vi "economizer exv valves.vi"(0 "Coarse Gas Input Cluster":T5={"Hot Gas Bypass\n Coarse Adjust"=100.0, "Accept Autotune Coarse Gas"=FALSE, "Coarse slide in P"=refnum, "file for Coarse gas"=path "", "autotune? Coarse gas"=FALSE, "PID gains in Coarse gas"={"proportional gain (Kc)"=0.0, "integral time (Ti, min)"=0.0, "derivative time (Td, min)"=0.0}} {"Hot Gas Bypass\n Coarse Adjust" min=0.0 max=100.0 step=1.0 scale=0.0..100.0}, 1 "Fine Gas Input Cluster":T6={"Hot Gas Bypass\n Fine Adjust"=100.0, "Accept Autotune Fine Gas"=FALSE, "Fine slide in P"=refnum, "file for fine gas"=path "", "autotune? fine gas"=FALSE, "PID gains in fine gas"={"proportional gain (Kc)"=0.0, "integral time (Ti, min)"=0.0, "derivative time (Td, min)"=0.0}} {"Hot Gas Bypass\n Fine Adjust" min=0.0 max=100.0 step=1.0 scale=0.0..100.0}, 3 "Intermediate T Threshold":dbl=5.0 format="%#_13g", 4 "Intermediate P Threshold":dbl=10.0 format="%#_13g", 5 "Coarse Liq Input Cluster":T3={"Liquid\n Coarse Adjust"=100.0, "Accept Autotune Coarse Liq"=FALSE, "Coarse slide in T"=refnum, "file for Coarse liq"=path "", "autotune? Coarse gas"=FALSE, "PID gains in Coarse Liq"={"proportional gain (Kc)"=0.0, "integral time (Ti, min)"=0.0, "derivative time (Td, min)"=0.0}} {"Liquid\n Coarse Adjust" min=0.0 max=100.0 step=1.0 scale=0.0..100.0}, 7 "Fine Liq Input Cluster":T4={"Liquid\n Fine Adjust"=100.0, "Accept Autotune Fine Liq"=FALSE, "Fine slide in T"=refnum, "file for fine liq"=path "", "autotune? fine liq"=FALSE, "PID gains in fine liq"={"proportional gain (Kc)"=0.0, "integral time (Ti, min)"=0.0, "derivative time (Td, min)"=0.0}} {"Liquid\n Fine Adjust" min=0.0 max=100.0 step=1.0 scale=0.0..100.0}, 8 "Controller Toggle P 2":bool, 9 "Reinitialize Controller P 2":bool, 10 "Economizer ?":bool, 12 "Current Intermediate T":dbl format="%#_13g", 13 "Desired Intermediate T":dbl, 14 "Desired Intermediate P":dbl, 15 "Current Intermediate P":dbl format="%#_13g", 16 "Controller Toggle T 2":bool, 17 "Reinitialize Controller T 2":bool) -> (20 "Gas Valves Output":T2, 27 "Liq Valves Output":T1)   [LabVIEW 2017]
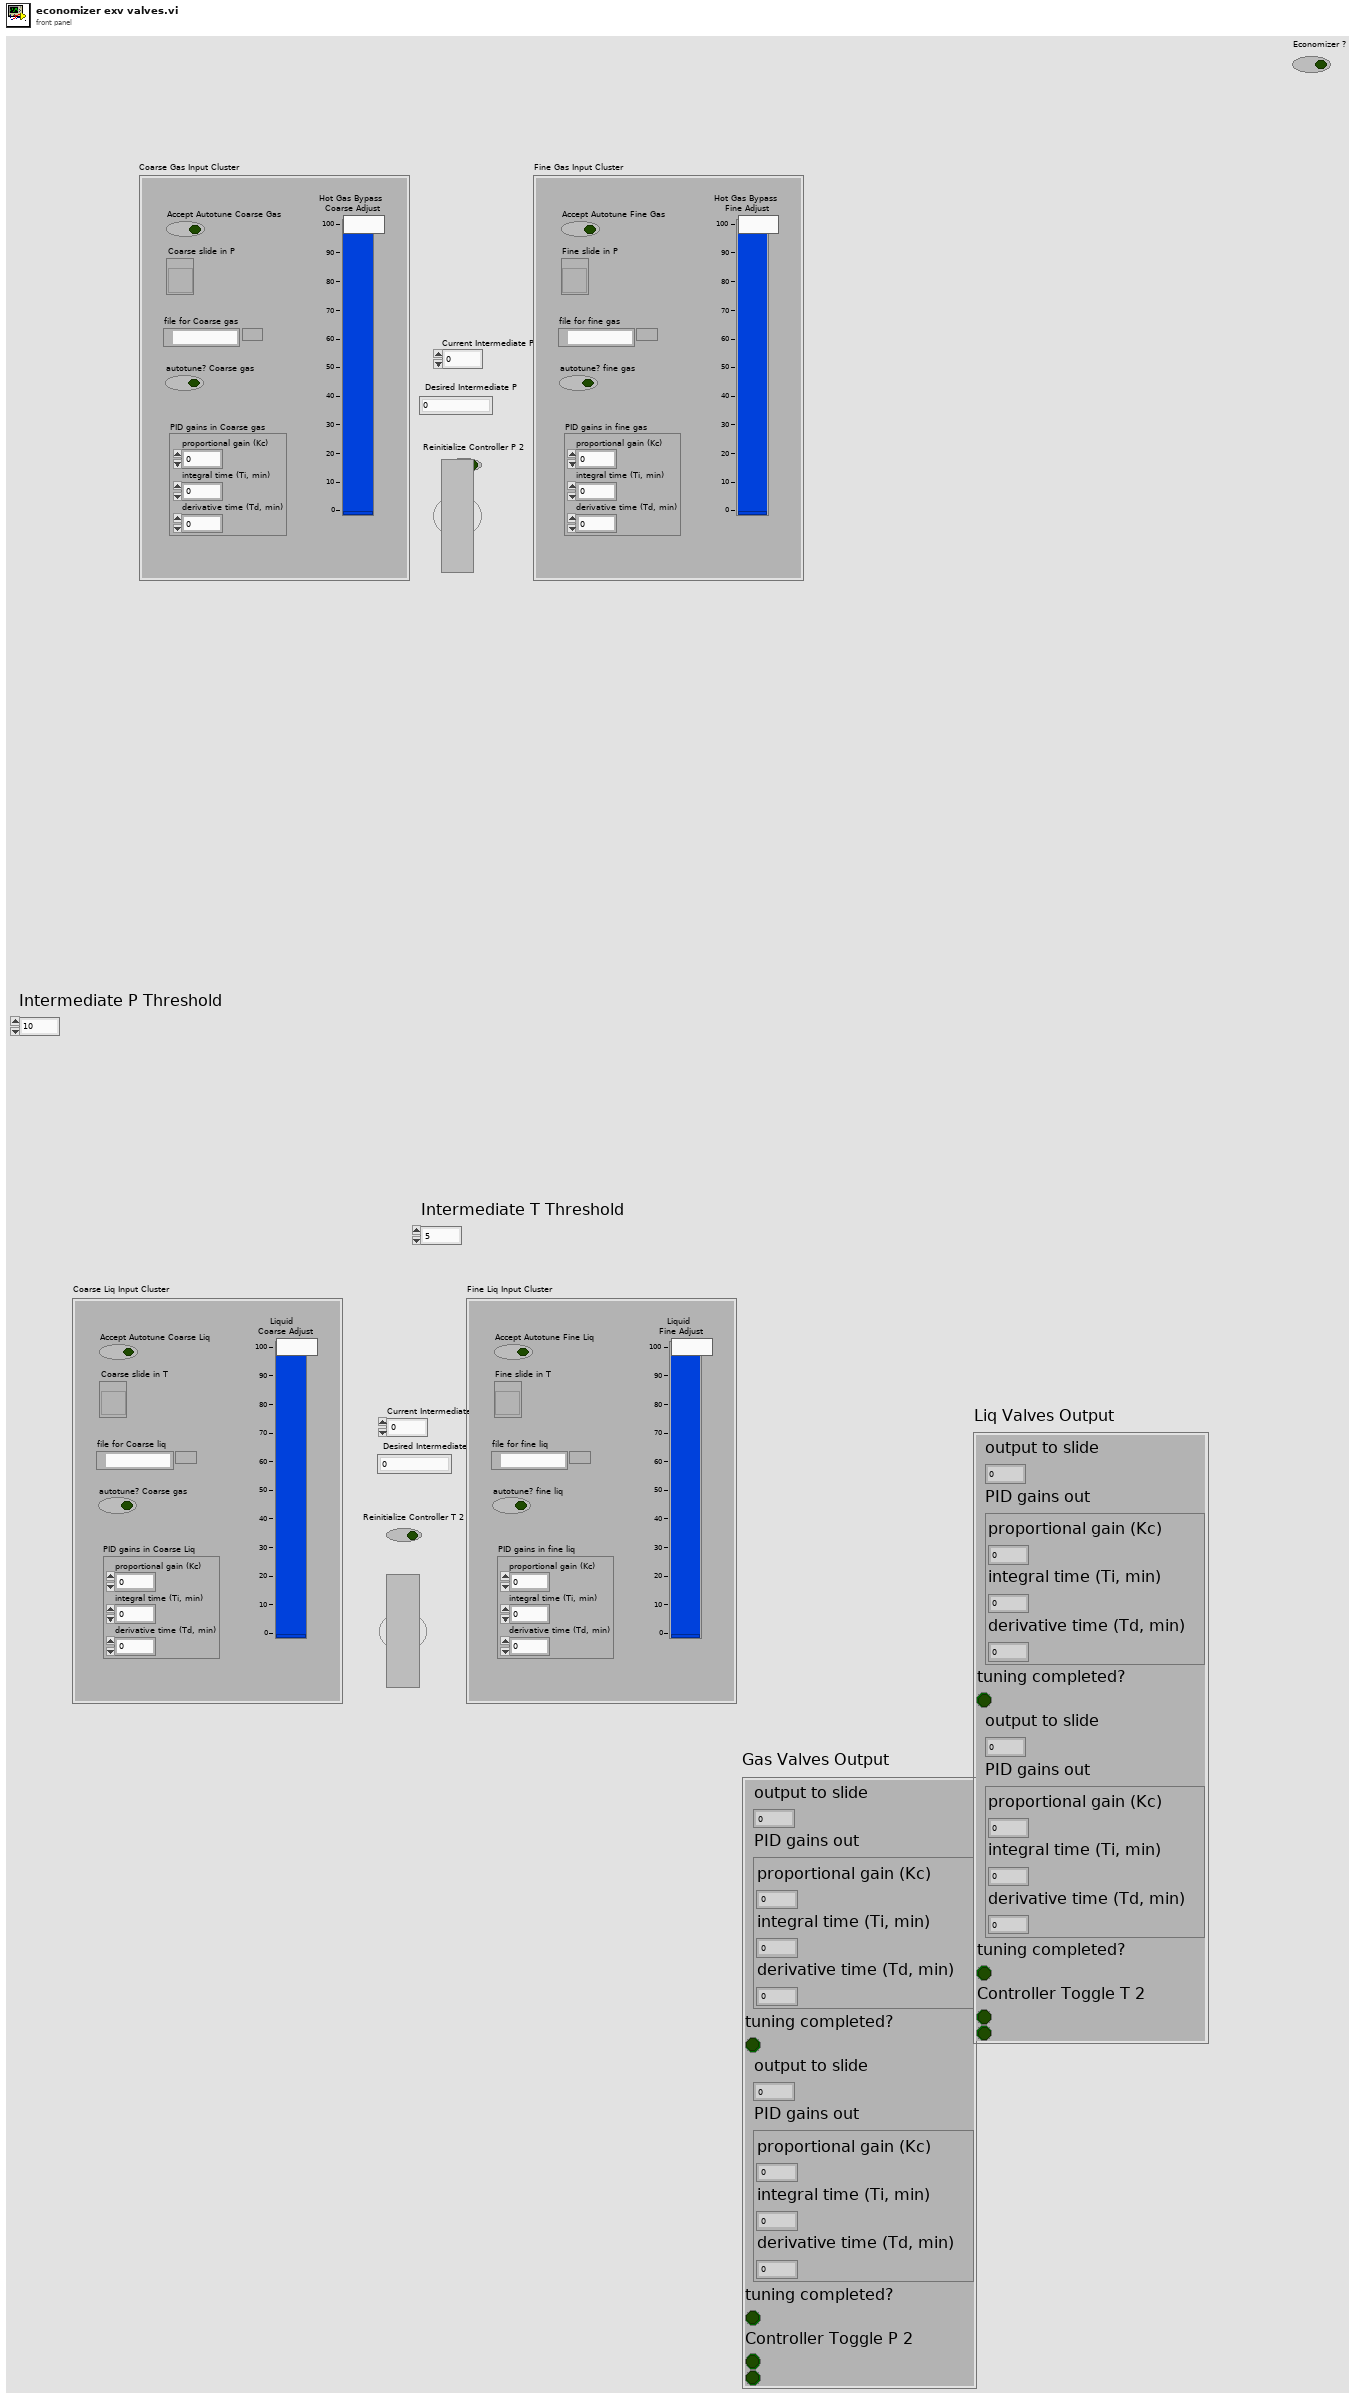
[diagram p1: front panel]
types:
  T1 = cluster{"output to slide":dbl, "PID gains out":cluster{"proportional gain (Kc)":dbl, "integral time (Ti, min)":dbl, "derivative time (Td, min)":dbl}, "tuning completed?":bool, "output to slide":dbl, "PID gains out":cluster{"proportional gain (Kc)":dbl, "integral time (Ti, min)":dbl, "derivative time (Td, min)":dbl}, "tuning completed?":bool, "Controller Toggle T 2":bool, bool}
  T2 = cluster{"output to slide":dbl, "PID gains out":cluster{"proportional gain (Kc)":dbl, "integral time (Ti, min)":dbl, "derivative time (Td, min)":dbl}, "tuning completed?":bool, "output to slide":dbl, "PID gains out":cluster{"proportional gain (Kc)":dbl, "integral time (Ti, min)":dbl, "derivative time (Td, min)":dbl}, "tuning completed?":bool, "Controller Toggle P 2":bool, bool}
  T3 = cluster{"Liquid\n Coarse Adjust":dbl, "Accept Autotune Coarse Liq":bool, "Coarse slide in T":refnum<vi>, "file for Coarse liq":path, "autotune? Coarse gas":bool, "PID gains in Coarse Liq":cluster{"proportional gain (Kc)":dbl, "integral time (Ti, min)":dbl, "derivative time (Td, min)":dbl}}
  T4 = cluster{"Liquid\n Fine Adjust":dbl, "Accept Autotune Fine Liq":bool, "Fine slide in T":refnum<vi>, "file for fine liq":path, "autotune? fine liq":bool, "PID gains in fine liq":cluster{"proportional gain (Kc)":dbl, "integral time (Ti, min)":dbl, "derivative time (Td, min)":dbl}}
  T5 = cluster{"Hot Gas Bypass\n Coarse Adjust":dbl, "Accept Autotune Coarse Gas":bool, "Coarse slide in P":refnum<vi>, "file for Coarse gas":path, "autotune? Coarse gas":bool, "PID gains in Coarse gas":cluster{"proportional gain (Kc)":dbl, "integral time (Ti, min)":dbl, "derivative time (Td, min)":dbl}}
  T6 = cluster{"Hot Gas Bypass\n Fine Adjust":dbl, "Accept Autotune Fine Gas":bool, "Fine slide in P":refnum<vi>, "file for fine gas":path, "autotune? fine gas":bool, "PID gains in fine gas":cluster{"proportional gain (Kc)":dbl, "integral time (Ti, min)":dbl, "derivative time (Td, min)":dbl}}
  T7 = cluster{"proportional gain (Kc)":dbl, "integral time (Ti, min)":dbl, "derivative time (Td, min)":dbl}
  T8 = enum8{"Enabled", "Disabled", "Disabled and Grayed Out"}
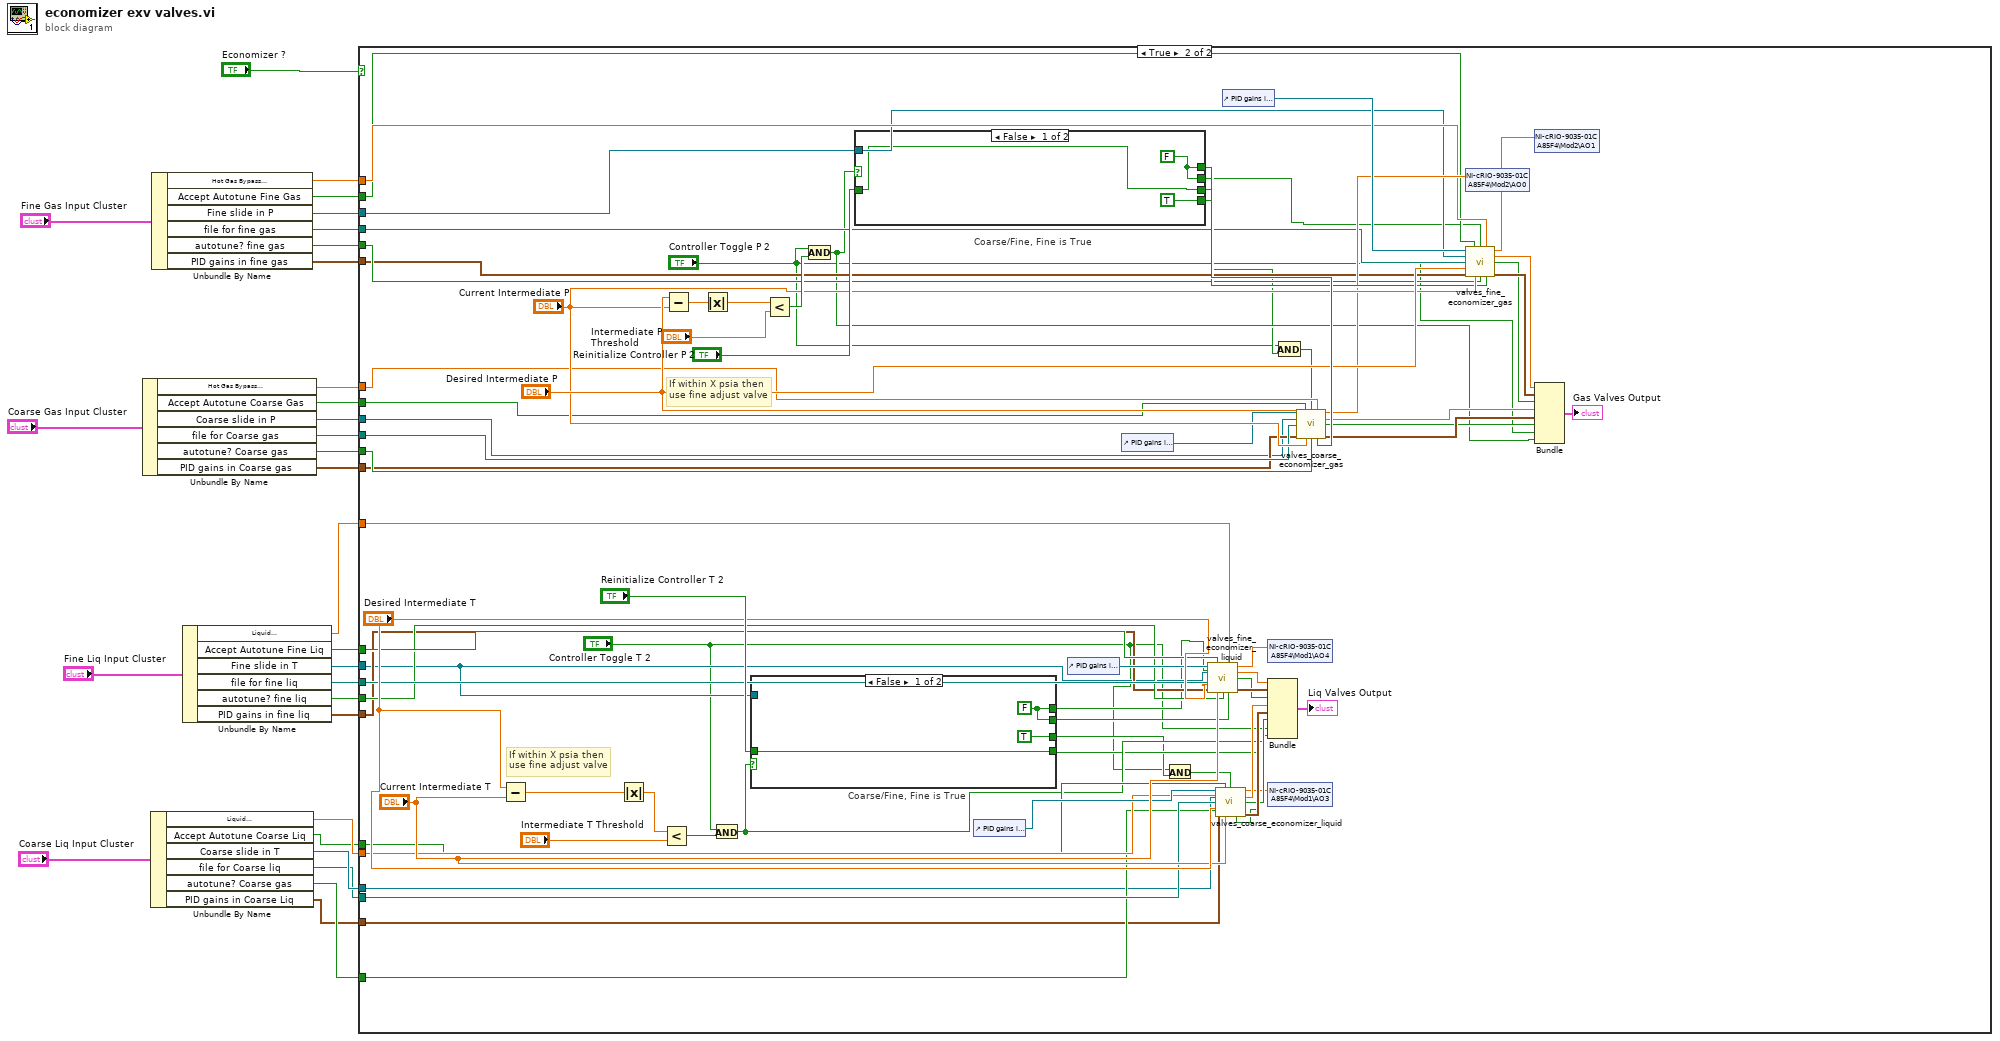
[diagram p0: block diagram]
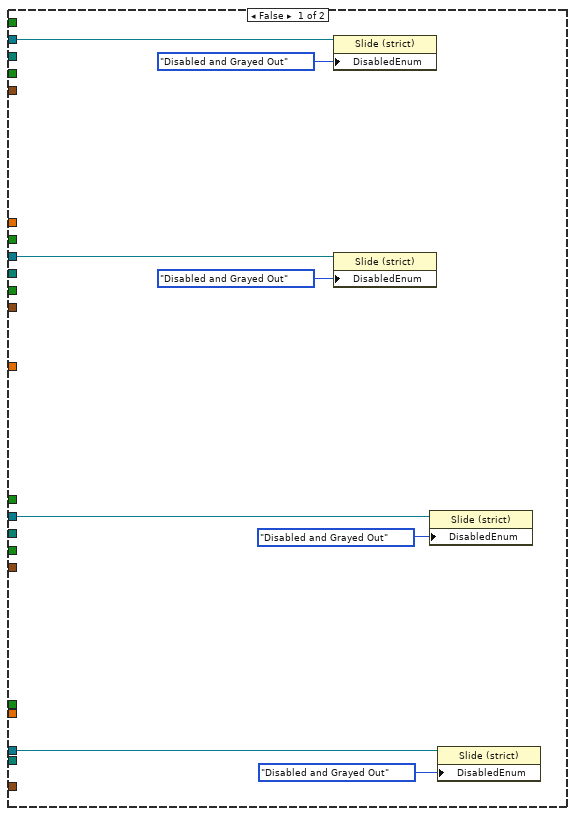
[diagram p2: hidden frame]
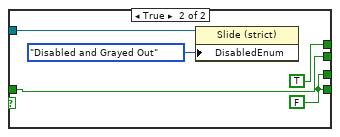
[diagram p3: hidden frame]
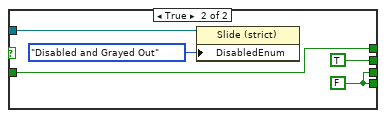
[diagram p4: hidden frame]
diagram:
  n1 = Unbundle By Name("Coarse Gas Input Cluster") -> ("Hot Gas Bypass\n Coarse Adjust"=w21:dbl, "Accept Autotune Coarse Gas"=w20:bool, "Coarse slide in P"=w19:refnum<vi>, "file for Coarse gas"=w18:path, "autotune? Coarse gas"=w17:bool, "PID gains in Coarse gas"=w16:T7)
  n2 = Unbundle By Name("Coarse Liq Input Cluster") -> ("Liquid\n Coarse Adjust"=w7:dbl, "Accept Autotune Coarse Liq"=w6:bool, "Coarse slide in T"=w5:refnum<vi>, "file for Coarse liq"=w4:path, "autotune? Coarse gas"=w3:bool, "PID gains in Coarse Liq"=w2:T7)
  n3 = Unbundle By Name("Fine Gas Input Cluster") -> ("Hot Gas Bypass\n Fine Adjust"=w28:dbl, "Accept Autotune Fine Gas"=w27:bool, "Fine slide in P"=w26:refnum<vi>, "file for fine gas"=w25:path, "autotune? fine gas"=w24:bool, "PID gains in fine gas"=w23:T7)
  n4 = Unbundle By Name("Fine Liq Input Cluster") -> ("Liquid\n Fine Adjust"=w14:dbl, "Accept Autotune Fine Liq"=w13:bool, "Fine slide in T"=w12:refnum<vi>, "file for fine liq"=w11:path, "autotune? fine liq"=w10:bool, "PID gains in fine liq"=w9:T7)
  n5 = case shown="True" "Economizer ?" {
    tunnel: w28 -> [_ w92]
    tunnel: w27 -> [_ w91]
    tunnel: w26 -> [w36 w47]
    tunnel: w25 -> [_ w90]
    tunnel: w24 -> [_ w89]
    tunnel: w23 -> [_ w88]
    tunnel: w21 -> [_ w87]
    tunnel: w20 -> [_ w86]
    tunnel: w19 -> [w34 w53]
    tunnel: w18 -> [_ w85]
    tunnel: w17 -> [_ w84]
    tunnel: w16 -> [_ w83]
    tunnel: w14 -> [_ w66]
    tunnel: w13 -> [_ w65]
    tunnel: w12 -> [w31 w48]
    tunnel: w11 -> [_ w64]
    tunnel: w10 -> [_ w63]
    tunnel: w9 -> [_ w62]
    tunnel: w7 -> [_ w61]
    tunnel: w6 -> [_ w60]
    tunnel: w5 -> [w30 w54]
    tunnel: w4 -> [_ w59]
    tunnel: w3 -> [_ w58]
    tunnel: w2 -> [_ w57]
    frame False {
      n6 = property on="Property Node" class="Slide (strict)"(reference=w36, "DisabledEnum"=T8."Disabled and Grayed Out" ("Disabled")) -> ()  [unwired: 1 in, 2 out]
      n7 = property on="Property Node" class="Slide (strict)"(reference=w34, "DisabledEnum"=T8."Disabled and Grayed Out" ("Disabled")) -> ()  [unwired: 1 in, 2 out]
      n8 = property on="Property Node" class="Slide (strict)"(reference=w31, "DisabledEnum"=T8."Disabled and Grayed Out" ("Disabled")) -> ()  [unwired: 1 in, 2 out]
      n9 = property on="Property Node" class="Slide (strict)"(reference=w30, "DisabledEnum"=T8."Disabled and Grayed Out" ("Disabled")) -> ()  [unwired: 1 in, 2 out]
    }
    frame True {
      # "If within X psia then\nuse fine adjust valve"
      # "If within X psia then\nuse fine adjust valve"
      n10 = Subtract(x="Desired Intermediate T", y="Current Intermediate T") -> (x-y=w82:dbl)
      n11 = Absolute Value(x=w82) -> (abs(x)=w81:dbl)
      n12 = Less?(x=w81, y="Intermediate T Threshold") -> (x < y?=w79:bool)
      n13 = Subtract(x="Desired Intermediate P", y="Current Intermediate P") -> (x-y=w111:dbl)
      n14 = Absolute Value(x=w111) -> (abs(x)=w110:dbl)
      n15 = And(x="Controller Toggle T 2", y=w79) -> (x .and. y?=w50:bool)
      n16 = case "Coarse/Fine, Fine is True" shown="False" w50 {
        tunnel: [w112 TRUE] -> w45
        tunnel: [TRUE w115] -> w43
        tunnel: "Reinitialize Controller T 2" -> [w113 w116]
        tunnel: [w112 w116] -> w75
        tunnel: [w113 w115] -> w46
        tunnel: w48 -> [_ w118]
        frame False {
          w112 = FALSE
        }
        frame True {
          w115 = FALSE
          n17 = property on="Property Node" class="Slide (strict)"(reference=w118, "DisabledEnum"=T8."Disabled and Grayed Out" ("Disabled")) -> ()  [unwired: 1 in, 2 out]
        }
      }
      n18 = Less?(x=w110, y="Intermediate P Threshold") -> (x < y?=w108:bool)
      n19 = And(x="Controller Toggle P 2", y=w108) -> (x .and. y?=w52:bool)
      n20 = case "Coarse/Fine, Fine is True" shown="False" w52 {
        tunnel: [w120 TRUE] -> w41
        tunnel: [TRUE w123] -> w39
        tunnel: "Reinitialize Controller P 2" -> [w121 w125]
        tunnel: [w120 w125] -> w103
        tunnel: [w121 w123] -> w106
        tunnel: w47 -> [_ w127]
        frame False {
          w120 = FALSE
        }
        frame True {
          w123 = FALSE
          n21 = property on="Property Node" class="Slide (strict)"(reference=w127, "DisabledEnum"=T8."Disabled and Grayed Out" ("Disabled")) -> ()  [unwired: 1 in, 2 out]
        }
      }
      n22 = control-ref of="PID gains in Coarse Liq"() -> (w73:refnum<vi>)
      n23 = control-ref of="PID gains in fine liq"() -> (w74:refnum<vi>)
      n24 = control-ref of="PID gains in Coarse gas"() -> (w101:refnum<vi>)
      n25 = And(x="Controller Toggle T 2", y=w43) -> (x .and. y?=w44:bool)
      n26 = call "valves_fine_economizer_liquid.vi"("PID Gains Cluster Ref"=w74, "Accept Autotune"=w65, "Controller Toggle (Manual Mode)"=w45, "Valve Manual Adjust"=w66, "Slide Refnum in"=w48, "file (use dialog)"=w64, "Desired Setpoint"="Desired Intermediate T", "PID gains"=w62, "Current Process Variable Value"="Current Intermediate T", "autotune? (F)"=w63, "Reinitialize Controller"=w75) -> ("output to valve"=w56:dbl, "output to slide"=w72:dbl, "tuning completed?"=w70:bool, "PID gains out"=w71:T7)  [unwired: 1 out]
      n27 = call "valves_coarse_economizer_liquid.vi"("PID Gains Cluster Ref"=w73, "Accept Autotune"=w60, "Controller Toggle (Manual Mode)"=w44, "Valve Manual Adjust"=w61, "Slide Refnum in"=w54, "file (use dialog)"=w59, "Desired Setpoint"="Desired Intermediate T", "PID gains"=w57, "Current Process Variable Value"="Current Intermediate T", "autotune? (F)"=w58, "Reinitialize Controller"=w46) -> ("output to valve"=w55:dbl, "output to slide"=w69:dbl, "tuning completed?"=w67:bool, "PID gains out"=w68:T7)  [unwired: 1 out]
      n28 = control-ref of="PID gains in fine gas"() -> (w102:refnum<vi>)
      n29 = shared-variable "NI-cRIO-9035-01CA85F4\\Mod1\\AO4"(w56) -> ()  [unwired: 1 in, 1 out]
      n30 = Bundle("output to slide"=w72, "PID gains out"=w71, "tuning completed?"=w70, "output to slide"=w69, "PID gains out"=w68, "tuning completed?"=w67, "Controller Toggle T 2"="Controller Toggle T 2", w50) -> (→"Liq Valves Output":T1)  [unwired: 1 in]
      n31 = shared-variable "NI-cRIO-9035-01CA85F4\\Mod1\\AO3"(w55) -> ()  [unwired: 1 in, 1 out]
      n32 = And(x="Controller Toggle P 2", y=w39) -> (x .and. y?=w40:bool)
      n33 = call "valves_coarse_economizer_gas.vi"("PID Gains Cluster Ref"=w101, "Accept Autotune"=w86, "Controller Toggle (Manual Mode)"=w40, "Valve Manual Adjust"=w87, "Slide Refnum in"=w53, "file (use dialog)"=w85, "Desired Setpoint"="Desired Intermediate P", "PID gains"=w83, "Current Process Variable Value"="Current Intermediate P", "autotune? (F)"=w84, "Reinitialize Controller"=w106) -> ("output to valve"=w94:dbl, "output to slide"=w97:dbl, "tuning completed?"=w95:bool, "PID gains out"=w96:T7)  [unwired: 1 out]
      n34 = shared-variable "NI-cRIO-9035-01CA85F4\\Mod2\\AO0"(w94) -> ()  [unwired: 1 in, 1 out]
      n35 = call "valves_fine_economizer_gas.vi"("PID Gains Cluster Ref"=w102, "Accept Autotune"=w91, "Controller Toggle (Manual Mode)"=w41, "Valve Manual Adjust"=w92, "Slide Refnum in"=w47, "file (use dialog)"=w90, "Desired Setpoint"="Desired Intermediate P", "PID gains"=w88, "Current Process Variable Value"="Current Intermediate P", "autotune? (F)"=w89, "Reinitialize Controller"=w103) -> ("output to valve"=w93:dbl, "output to slide"=w100:dbl, "tuning completed?"=w98:bool, "PID gains out"=w99:T7)  [unwired: 1 out]
      n36 = shared-variable "NI-cRIO-9035-01CA85F4\\Mod2\\AO1"(w93) -> ()  [unwired: 1 in, 1 out]
      n37 = Bundle("output to slide"=w100, "PID gains out"=w99, "tuning completed?"=w98, "output to slide"=w97, "PID gains out"=w96, "tuning completed?"=w95, "Controller Toggle P 2"="Controller Toggle P 2", w52) -> (→"Gas Valves Output":T2)  [unwired: 1 in]
    }
  }
